vi "Launcher.vi"() -> ()   [LabVIEW 2012]
uses:
  StateMachineEnum.ctl
  Robot Global Data.vi
panel:
  out "Loop interval (ms)":u32
  in  "PID R":T1={"proportional gain (Kc)"=0.0008, "integral time (Ti, min)"=0.010000000000000009, "derivative time (Td, min)"=0.0} {"derivative time (Td, min)" step=0.01 format="%.2f"; "integral time (Ti, min)" step=0.01 format="%.2f"; "proportional gain (Kc)" step=0.0001 format="%.4f"}
  in  "Output R":cluster{"output high":dbl, "output low":dbl}={"output high"=1.0, "output low"=0.0} {"output low" step=0.1 format="%.2f"; "output high" step=0.1 format="%.2f"}
  in  "PID L":T1={"proportional gain (Kc)"=0.0008, "integral time (Ti, min)"=0.01, "derivative time (Td, min)"=0.0} {"derivative time (Td, min)" step=0.01 format="%.2f"; "integral time (Ti, min)" step=0.01 format="%.2f"; "proportional gain (Kc)" step=0.0001 format="%.4f"}
  in  "Output L":cluster{"output high":dbl, "output low":dbl}={"output high"=1.0, "output low"=0.0} {"output low" step=0.1 format="%.2f"; "output high" step=0.1 format="%.2f"}
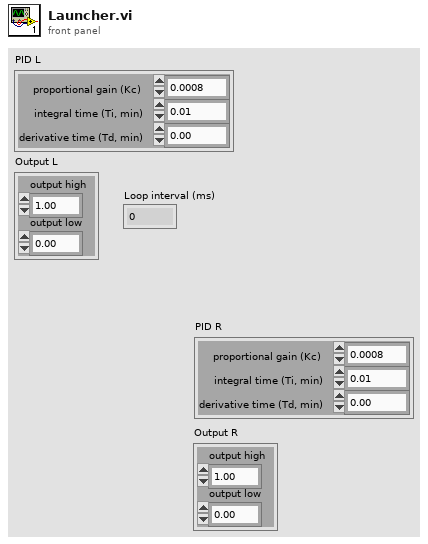
[diagram p1: front panel]
types:
  T1 = cluster{"proportional gain (Kc)":dbl, "integral time (Ti, min)":dbl, "derivative time (Td, min)":dbl}
  T2 = typedef "StateMachineEnum.ctl" = enum16{"Init", "Idle", "Start", "Do", "Stop"}
  T3 = typedef "WPI_MotorControlDeviceRef.ctl" = cluster{"DeviceStatus":errorcluster, "Type":enum16{"PWM", "CAN"}, "PWM":cluster{"Digital Module":T4, "PWM Channel":T5, "DeadBand":T6}, "CAN":cluster{"Device Number":u8, "Control Mode":T7, "Semaphore":T8, "Max Vout":dbl}, "Invert":bool, "TransformRef":T9, "InvTransformRef":T9}
  T4 = typedef "FPGA_TypedefDigitalModule.ctl" = enum16{"Digital Module 1", "Digital Module 2"}
  T5 = typedef "FPGA_DIOPWMChannel.ctl" = enum8{"PWM 1", "PWM 2", "PWM 3", "PWM 4", "PWM 5", "PWM 6", "PWM 7", "PWM 8", "PWM 9", "PWM 10", "Invalid"}
  T6 = typedef "WPI_PWMDeadband.ctl" = cluster{"Name":string, "maxPositivePwm":i32, "minPositivePwm":i32, "centerPwm":i32, "maxNegativePwm":i32, "minNegativePwm":i32, "angularRange":u16}
  T7 = typedef "WPI_CANJaguar_ControlMode.ctl" = enum8{"Percent VBus", "Current", "Speed", "Position", "Voltage"}
  T8 = typedef "Semaphore RefNum" = refnum<k1>
  T9 = typedef "WPI_PWMTransform_ConPane.ctl" = refnum<vi>
  T10 = typedef "WPI_CounterDevRef.ctl" = cluster{"DevStatus":errorcluster, "CntIndex":T11}
  T11 = typedef "FPGA_CounterCtrSystemIndex.ctl" = enum8{"Ctr 0", "Ctr 1", "Ctr 2", "Ctr 3", "Ctr 4", "Ctr 5", "Ctr 6", "Ctr 7", "Invalid"}
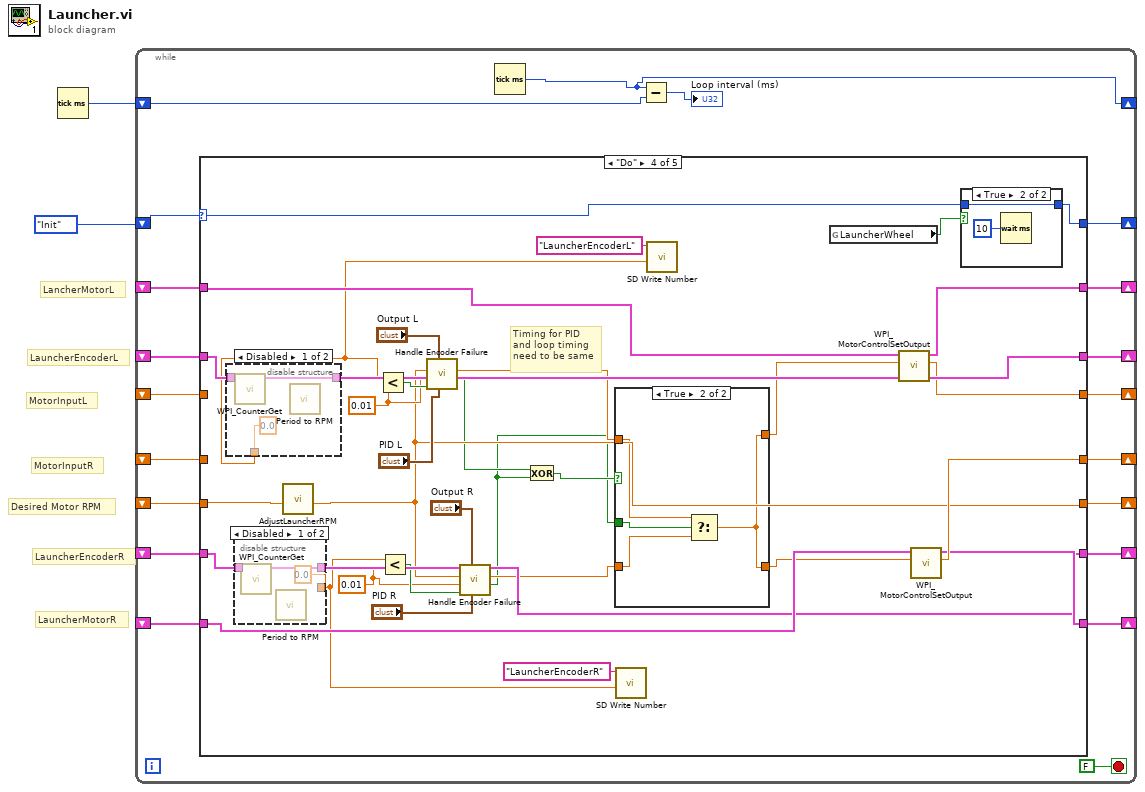
[diagram p0: block diagram]
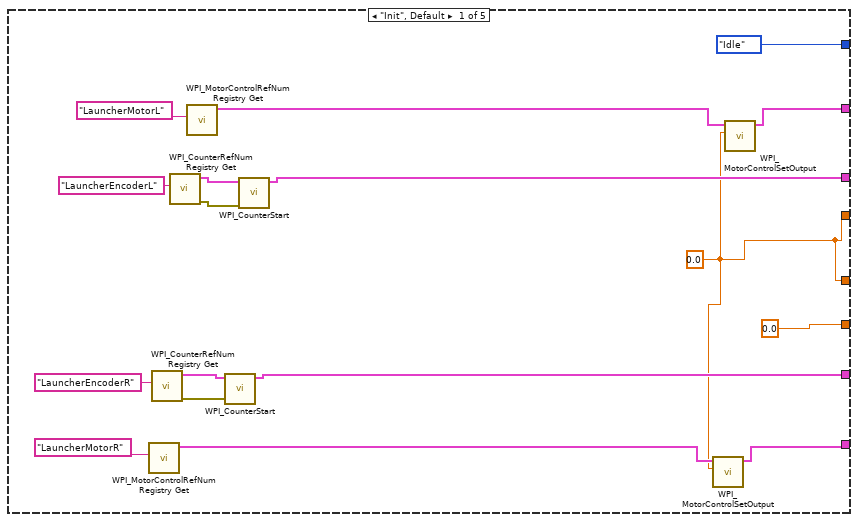
[diagram p2: hidden frame]
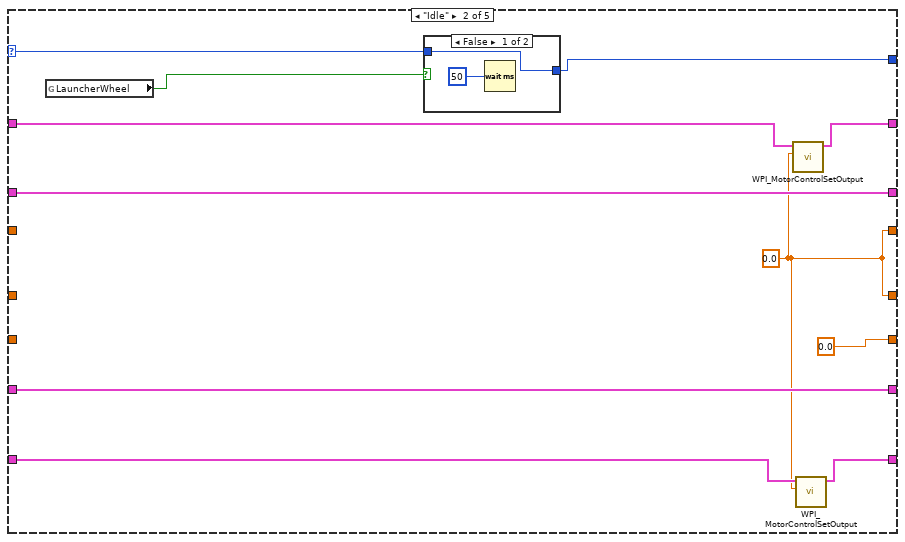
[diagram p3: hidden frame]
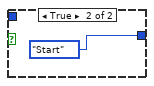
[diagram p4: hidden frame]
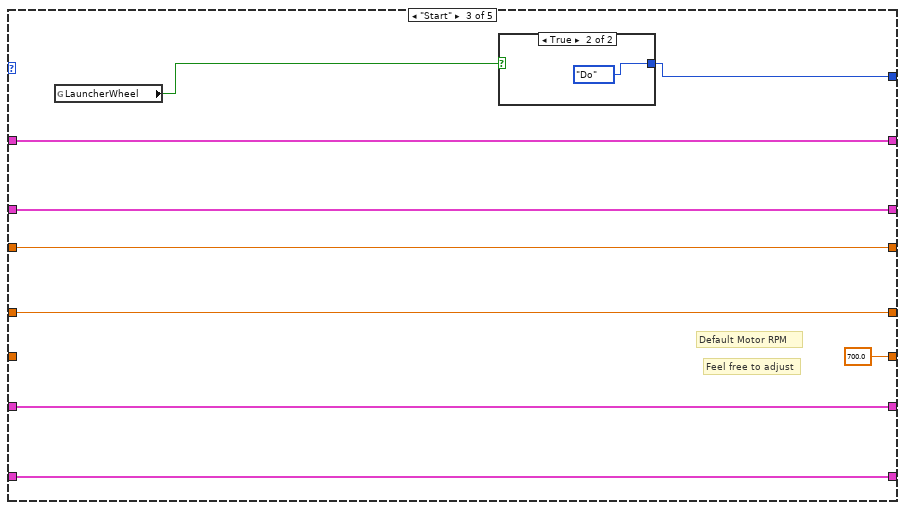
[diagram p5: hidden frame]
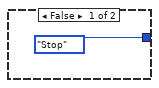
[diagram p6: hidden frame]
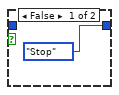
[diagram p10: hidden frame]
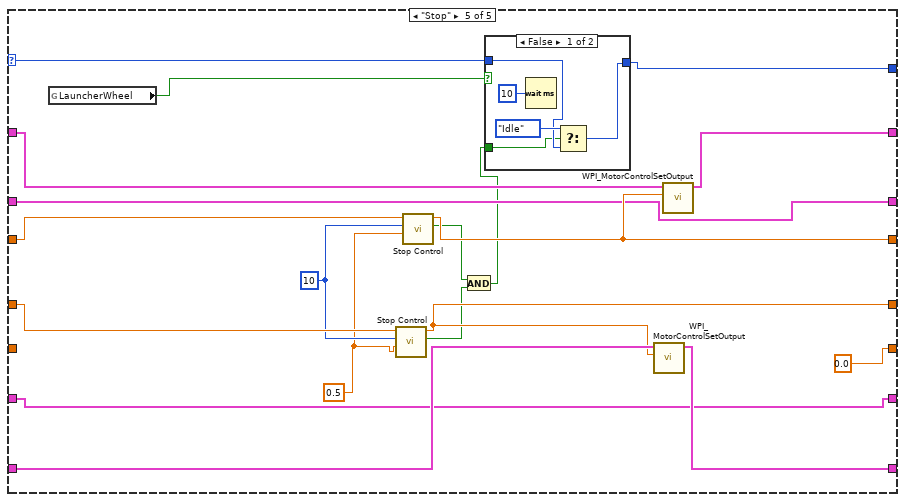
[diagram p11: hidden frame]
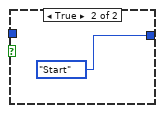
[diagram p12: hidden frame]
diagram:
  # "Desired Motor RPM"
  # "MotorInputR"
  # "MotorInputL"
  # "LauncherMotorR"
  # "LauncherEncoderR"
  # "LauncherEncoderL"
  # "LancherMotorL"
  n1 = Tick Count (ms)() -> (millisecond timer value=w1:u32)
  n2 = while {
    shift-right: [w21] -> _
    shift-left: _ -> [w11]
    shift-right: [w20] -> _
    shift-left: _ -> [w12]
    shift-right: [w19] -> _
    shift-left: _ -> [w10]
    shift-right: [w18] -> _
    shift-left: _ -> [w9]
    shift-right: [w17] -> _
    shift-left: StateMachineEnum."Init" ("State") -> [w22]
    shift-right: [w16] -> _
    shift-left: _ -> [w14]
    shift-right: [w15] -> _
    shift-left: _ -> [w13]
    shift-right: [w7] -> _
    shift-left: _ -> [w6]
    shift-right: [w3] -> _
    shift-left: w1 -> [w4]
    stop <- FALSE stop-if-true
    n3 = case shown="\"Do\"" w22 {
      selector: w22 -> [_ w49 _ w97 w131]
      tunnel: [w27 w44 w60 w90 w124] -> w21
      tunnel: [w29 w47 w59 w87 w123] -> w20
      tunnel: [w33 w46 w58 w88 w119] -> w19
      tunnel: [w25 w42 w57 w89 w120] -> w18
      tunnel: [StateMachineEnum."Idle" ("State") w48 w61 w96 w130] -> w17
      tunnel: [w24 w41 w56 w86 w125] -> w16
      tunnel: [w24 w41 w55 w91 w121] -> w15
      tunnel: w14 -> [_ _ w56 _ w129]
      tunnel: w13 -> [_ _ w55 _ w128]
      tunnel: w12 -> [_ w47 w59 w95 w123]
      tunnel: w11 -> [_ w45 w60 w92 w126]
      tunnel: w10 -> [_ w46 w58 w94 w119]
      tunnel: w9 -> [_ w43 w57 w93 w122]
      tunnel: [0.0 ("y") 0.0 ("y") 700.0 w76 0.0 ("y")] -> w7
      tunnel: w6 -> [_ _ _ w85 _]
      frame "Init", Default {
        w24 = 0.0
        n4 = call <vilib>:"WPI_MotorControlRefNum Registry Get.vi"("refnum name"="LauncherMotorR") -> ("MotorControlDevRef"=w26:T3)  [unwired: 9 in, 1 out]
        n5 = call <vilib>:"WPI_CounterRefNum Registry Get.vi"("refnum name"="LauncherEncoderR") -> ("error out"=w32:errorcluster, "CounterDevRef"=w34:T10)  [unwired: 9 in]
        n6 = call <vilib>:"WPI_CounterRefNum Registry Get.vi"("refnum name"="LauncherEncoderL") -> ("error out"=w30:errorcluster, "CounterDevRef"=w31:T10)  [unwired: 9 in]
        n7 = call <vilib>:"WPI_MotorControlRefNum Registry Get.vi"("refnum name"="LauncherMotorL") -> ("MotorControlDevRef"=w28:T3)  [unwired: 9 in, 1 out]
        n8 = call <vilib>:"WPI_CounterStart.vi"("error in (no error)"=w32, "CounterDevRef in"=w34) -> ("CounterDevRef out"=w33:T10)  [unwired: 8 in, 1 out]
        n9 = call <vilib>:"WPI_CounterStart.vi"("error in (no error)"=w30, "CounterDevRef in"=w31) -> ("CounterDevRef out"=w29:T10)  [unwired: 8 in, 1 out]
        n10 = call <vilib>:"WPI_MotorControlSetOutput.vi"("Output"=w24, "MotorControlDevRef"=w26) -> ("MotorControlDevRef"=w25:T3)  [unwired: 7 in, 2 out]
        n11 = call <vilib>:"WPI_MotorControlSetOutput.vi"("Output"=w24, "MotorControlDevRef"=w28) -> ("MotorControlDevRef"=w27:T3)  [unwired: 7 in, 2 out]
      }
      frame "Idle" {
        w41 = 0.0
        n12 = global read "Robot Global Data.vi" "LauncherWheel"() -> (w50:bool)
        n13 = case shown="False" w50 {
          tunnel: w49 -> [w52 _]
          tunnel: [w52 StateMachineEnum."Start" ("State")] -> w48
          frame False {
            n14 = Wait (ms)(milliseconds to wait=u32 50) -> ()  [unwired: 1 out]
          }
          frame True {
          }
        }
        n15 = call <vilib>:"WPI_MotorControlSetOutput.vi"("Output"=w41, "MotorControlDevRef"=w45) -> ("MotorControlDevRef"=w44:T3)  [unwired: 7 in, 2 out]
        n16 = call <vilib>:"WPI_MotorControlSetOutput.vi"("Output"=w41, "MotorControlDevRef"=w43) -> ("MotorControlDevRef"=w42:T3)  [unwired: 7 in, 2 out]
      }
      frame "Start" {
        # "Feel free to adjust"
        # "Default Motor RPM"
        n17 = global read "Robot Global Data.vi" "LauncherWheel"() -> (w62:bool)
        n18 = case shown="True" w62 {
          tunnel: [StateMachineEnum."Stop" ("State") StateMachineEnum."Do" ("State")] -> w61
          frame False {
          }
          frame True {
          }
        }
      }
      frame "Do" {
        w77 = 0.01
        w81 = 0.01
        # "Timing for PID\nand loop timing\nneed to be same"
        n19 = disable-structure shown="Disabled" {
          disable-tunnel: [0.0 ("Period (sec)") _] -> w66
          disable-tunnel: w95 -> [w104 _]
          disable-tunnel: [w103 _] -> w87
          frame Disabled {
            n20 = call <vilib>:"WPI_CounterGet.vi"("CounterDevRef in"=w104) -> ("CounterDevRef out"=w103:T10)  [unwired: 5 in, 5 out]
            n21 = call "Period to RPM.vi"() -> ()  [unwired: 11 in, 1 out]
          }
          frame Enabled {
          }
        }
        n22 = disable-structure shown="Disabled" {
          disable-tunnel: [0.0 ("Period (sec)") _] -> w65
          disable-tunnel: w94 -> [w101 _]
          disable-tunnel: [w100 _] -> w88
          frame Disabled {
            n23 = call <vilib>:"WPI_CounterGet.vi"("CounterDevRef in"=w101) -> ("CounterDevRef out"=w100:T10)  [unwired: 5 in, 5 out]
            n24 = call "Period to RPM.vi"() -> ()  [unwired: 11 in, 1 out]
          }
          frame Enabled {
          }
        }
        n25 = call "AdjustLauncherRPM.vi"("Current RPM"=w85) -> ("New RPM"=w76:dbl)  [unwired: 10 in]
        n26 = Less?(x=w66, y=w77) -> (x < y?=w78:bool)
        n27 = Less?(x=w65, y=w81) -> (x < y?=w82:bool)
        n28 = call "Handle Encoder Failure.vi"("PID gains"="PID L", "Output Range"="Output L", "Encoder Failure"=w78, "Loop Time"=w77, "Desired RPM"=w76) -> ("Encoder Failure Out"=w70:bool, "Motor Output"=w74:dbl)  [unwired: 5 in]
        n29 = call "Handle Encoder Failure.vi"("PID gains"="PID R", "Output Range"="Output R", "Encoder Failure"=w82, "Loop Time"=w81, "Desired RPM"=w76) -> ("Encoder Failure Out"=w69:bool, "Motor Output"=w73:dbl)  [unwired: 5 in]
        n30 = Exclusive Or(1:w69, 2:w70) -> (0:w75:bool)
        n31 = case shown="True" w75 {
          tunnel: w74 -> [w106 w108]
          tunnel: w73 -> [w105 w109]
          tunnel: [w105 w107] -> w72
          tunnel: [w106 w107] -> w71
          tunnel: w69 -> [_ w110]
          frame False {
          }
          frame True {
            n32 = Select(t=w108, s=w110, f=w109) -> (s? t:f=w107:dbl)
          }
        }
        n33 = call <vilib>:"SD Write Number.vi"("Numeric"=w65, "Name"="LauncherEncoderR") -> ()  [unwired: 8 in, 2 out]
        n34 = call <vilib>:"SD Write Number.vi"("Numeric"=w66, "Name"="LauncherEncoderL") -> ()  [unwired: 8 in, 2 out]
        n35 = global read "Robot Global Data.vi" "LauncherWheel"() -> (w98:bool)
        n36 = call <vilib>:"WPI_MotorControlSetOutput.vi"("Output"=w71, "MotorControlDevRef"=w92) -> ("Motor Output"=w86:dbl, "MotorControlDevRef"=w90:T3)  [unwired: 7 in, 1 out]
        n37 = call <vilib>:"WPI_MotorControlSetOutput.vi"("Output"=w72, "MotorControlDevRef"=w93) -> ("Motor Output"=w91:dbl, "MotorControlDevRef"=w89:T3)  [unwired: 7 in, 1 out]
        n38 = case shown="True" w98 {
          tunnel: w97 -> [_ w112]
          tunnel: [StateMachineEnum."Stop" ("State") w112] -> w96
          frame False {
          }
          frame True {
            n39 = Wait (ms)(milliseconds to wait=u32 10) -> ()  [unwired: 1 out]
          }
        }
      }
      frame "Stop" {
        w115 = 0.5 ("y")
        w127 = u32 10 ("milliseconds to wait")
        n40 = global read "Robot Global Data.vi" "LauncherWheel"() -> (w132:bool)
        n41 = call "Stop Control.vi"("Rate (unit/s)"=w115, "Loop Time (ms)"=w127, "Recieved Motor Input"=w128) -> ("Done Stopping"=w117:bool, "New Motor Input"=w121:dbl)  [unwired: 7 in]
        n42 = call "Stop Control.vi"("Rate (unit/s)"=w115, "Loop Time (ms)"=w127, "Recieved Motor Input"=w129) -> ("Done Stopping"=w118:bool, "New Motor Input"=w125:dbl)  [unwired: 7 in]
        n43 = And(x=w118, y=w117) -> (x .and. y?=w116:bool)
        n44 = case shown="False" w132 {
          tunnel: w131 -> [w135 _]
          tunnel: [w134 StateMachineEnum."Start" ("State")] -> w130
          tunnel: w116 -> [w133 _]
          frame False {
            n45 = Wait (ms)(milliseconds to wait=u32 10) -> ()  [unwired: 1 out]
            n46 = Select(t=StateMachineEnum."Idle" ("State"), s=w133, f=w135) -> (s? t:f=w134:T2)
          }
          frame True {
          }
        }
        n47 = call <vilib>:"WPI_MotorControlSetOutput.vi"("Output"=w121, "MotorControlDevRef"=w122) -> ("MotorControlDevRef"=w120:T3)  [unwired: 7 in, 2 out]
        n48 = call <vilib>:"WPI_MotorControlSetOutput.vi"("Output"=w125, "MotorControlDevRef"=w126) -> ("MotorControlDevRef"=w124:T3)  [unwired: 7 in, 2 out]
      }
    }
    n49 = Tick Count (ms)() -> (millisecond timer value=w3:u32)
    n50 = Subtract(x=w3, y=w4) -> (x-y=→"Loop interval (ms)":u32)
  }
